vi "Negate Color.vi"(11 "image data in":T1) -> (3 "image data out":T1)   [LabVIEW 2017]
uses:
  <vilib>/picture/picture.llb/imagedata.ctl
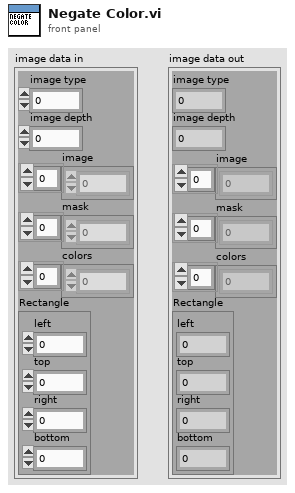
[diagram p1: front panel]
types:
  T1 = typedef "imagedata.ctl" = cluster{"image type":i32, "image depth":i32, "image":u8[], "mask":u8[], "colors":u32[], "Rectangle":cluster{"left":i16, "top":i16, "right":i16, "bottom":i16}}
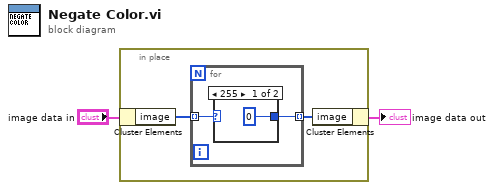
[diagram p0: block diagram]
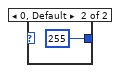
[diagram p2: hidden frame]
diagram:
  n1 = in-place {
    n2 = in-place-cluster #1("image data in") -> ("image"=w4:u8[])
    n3 = for {
      tunnel: w4 -> [w6] mode=indexing
      tunnel: [w5] -> w3 mode=indexing
      n4 = case shown="255" w6 {
        tunnel: [u8 0 u8 255] -> w5
        frame 255 {
        }
        frame 0, Default {
        }
      }
    }
    n5 = in-place-cluster #1("image"=w3) -> (→"image data out":T1)
  }
